vi "main.vi"() -> ()   [LabVIEW 2024]
uses:
  controls/adam-module-select-tab.ctl
  controls/digital-output-cluster.ctl
  controls/digitial-input-cluster.ctl
  controls/analog-output-cluster.ctl
  controls/analog-input-cluster.ctl
  controls/thermocouple-input-cluster.ctl
  controls/adam-5000-serial-settings.ctl
  controls/state-enum.ctl
  <vilib>/Instr/_visa.llb/VISA Configure Serial Port (Instr).vi
  <vilib>/Instr/_visa.llb/VISA Flush IO Buffer Mask.ctl
panel:
  out "response":string
  out "cmd string":string
  out "Ack":bool
  out "Sampling":bool
  in  "Module Type":T1(ring)
  out "slot: 0":T2
  in  "Digital Outputs":T3
  out "Digital Inputs":T4
  in  "Analog Outputs":T5
  out "Analog Inputs":T6
  out "Thermocouple Inputs (degC)":T7
  in  "Chassis Settings":T8={"VISA resource name"="COM10", "baud rate (19200)"=19200, "Chassis ID"=1}
  in  "Debug Mode":bool
  out "Loop Time (mS)":u32
  out "Loop Counter":i32
  out "Write Success":bool
  out "error IO":errorcluster
  out "error":errorcluster
  in  "exit":bool
  # "ADAM 5000 Controller"
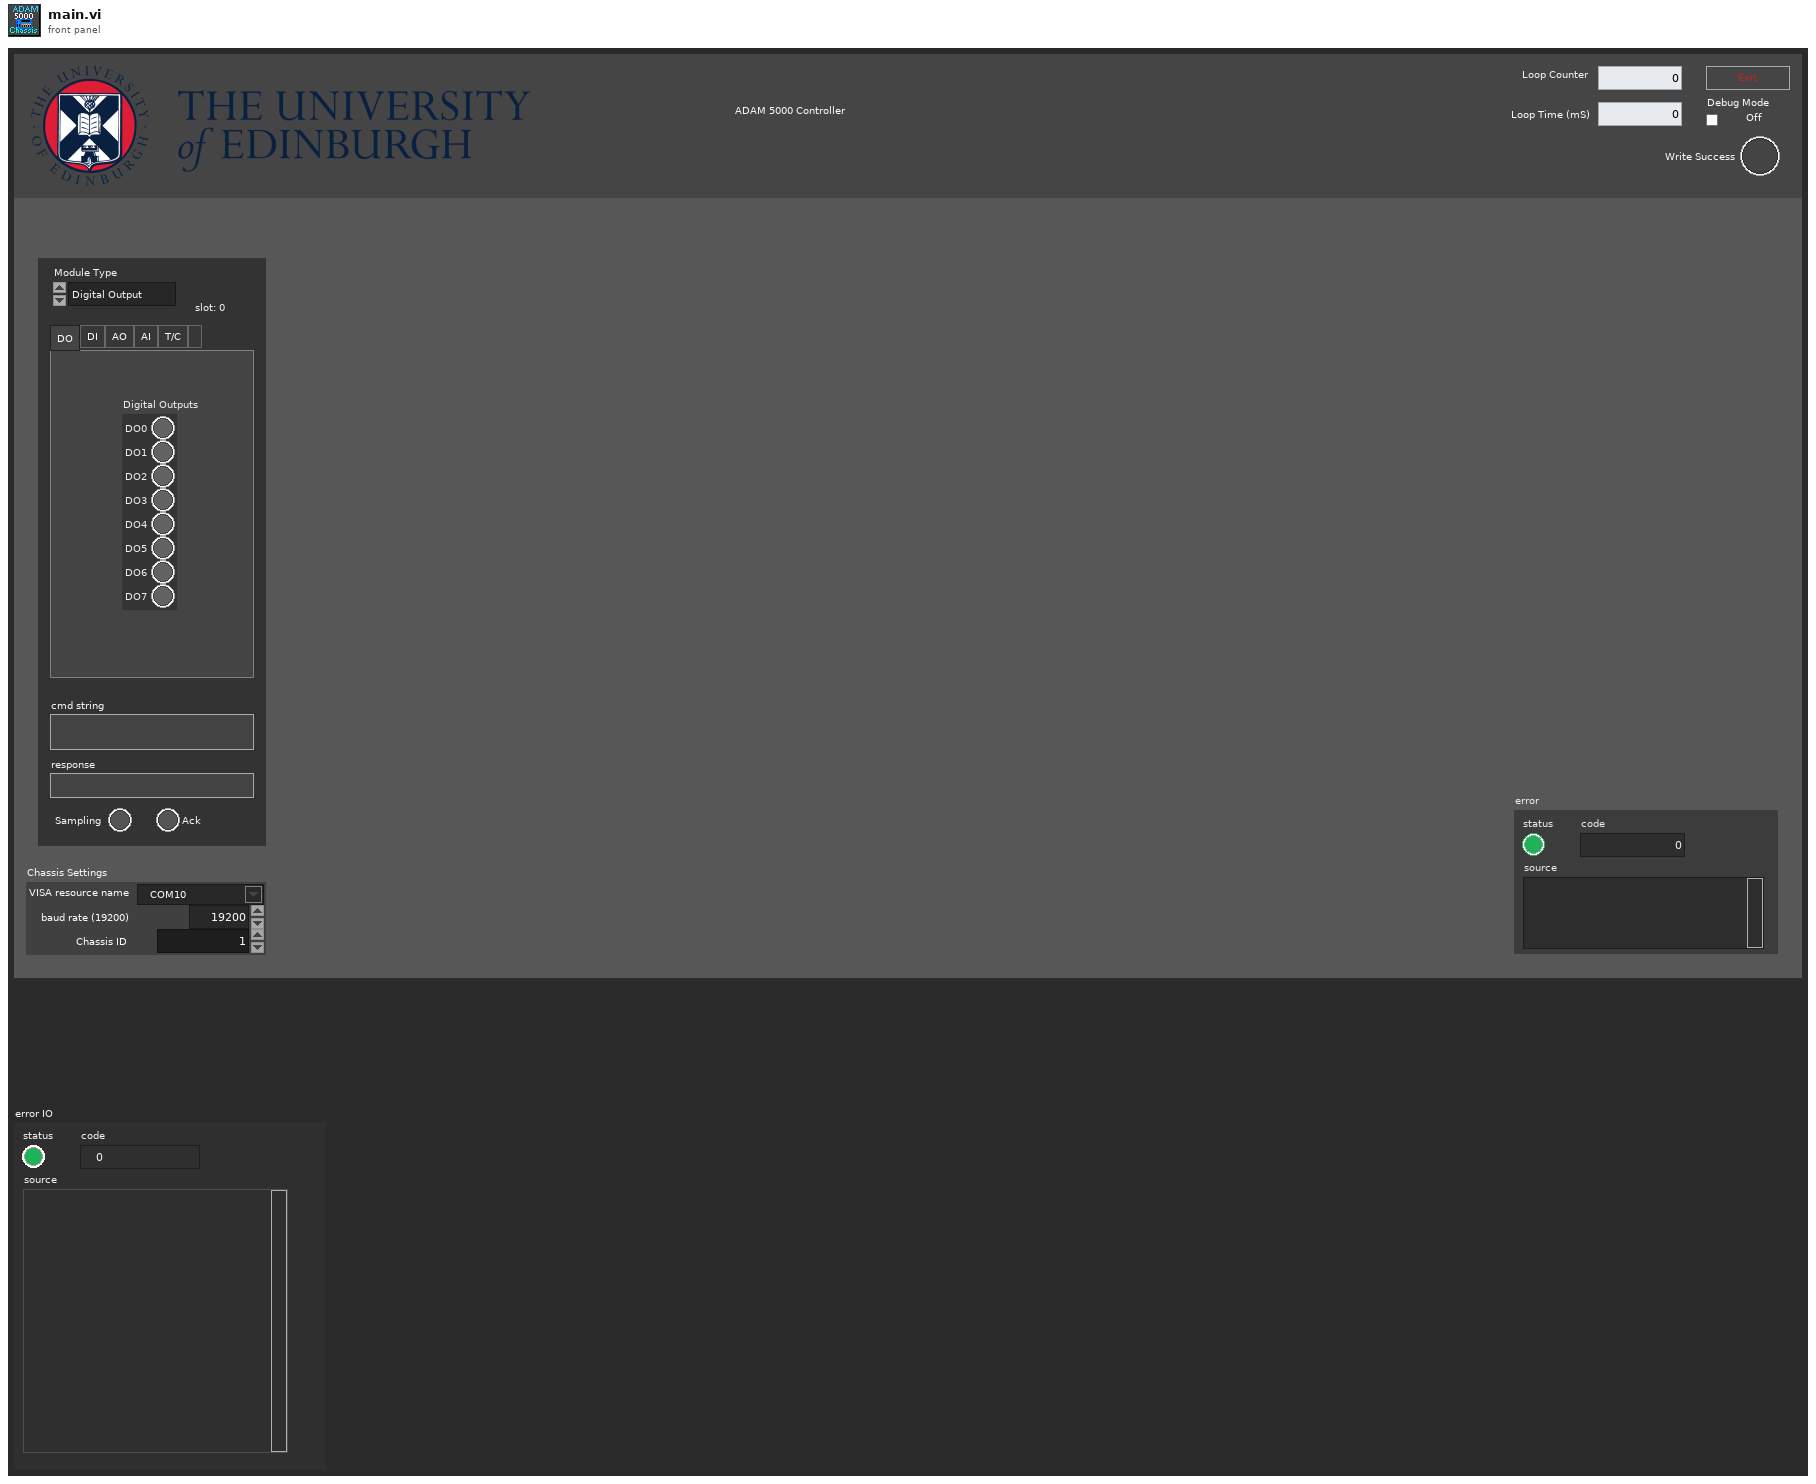
[diagram p1: front panel]
types:
  T1 = enum16{"Digital Output", "Digital Input", "Analog Output", "Analog Input", "Thermocouple", "Power Relay", "empty"}
  T2 = typedef "adam-module-select-tab.ctl" = enum32{"DO", "DI", "AO", "AI", "T/C", ""}
  T3 = typedef "digital-output-cluster.ctl" = cluster{"DO0":bool, "DO1":bool, "DO2":bool, "DO3":bool, "DO4":bool, "DO5":bool, "DO6":bool, "DO7":bool}
  T4 = typedef "digitial-input-cluster.ctl" = cluster{"DI0":bool, "DI1":bool, "DI2":bool, "DI3":bool, "DI4":bool, "DI5":bool, "DI6":bool, "DI7":bool}
  T5 = typedef "analog-output-cluster.ctl" = cluster{"AO0":dbl, "AO1":dbl, "AO2":dbl, "AO3":dbl, "AO4":dbl, "AO5":dbl, "AO6":dbl, "AO7":dbl}
  T6 = typedef "analog-input-cluster.ctl" = cluster{"AO0":dbl, "AO1":dbl, "AO2":dbl, "AO3":dbl, "AO4":dbl, "AO5":dbl, "AO6":dbl, "AO7":dbl}
  T7 = typedef "thermocouple-input-cluster.ctl" = cluster{"TC0":dbl, "TC1":dbl, "TC2":dbl, "TC3":dbl, "TC4":dbl, "TC5":dbl, "TC6":dbl}
  T8 = typedef "adam-5000-serial-settings.ctl" = cluster{"VISA resource name":refnum<visa-resource-name>, "baud rate (19200)":u32, "Chassis ID":u8}
  T9 = cluster{"Digital Outputs":T3, "Digital Inputs":T4, "Analog Outputs":T5, "Analog Inputs":T6, "Thermocouple Inputs (degC)":T7}
  T10 = typedef "state-enum.ctl" = enum16{"init", "manual", "start", "run", "hold", "stop", ""}
  T11 = typedef "VISA Flush IO Buffer Mask.ctl" = u16
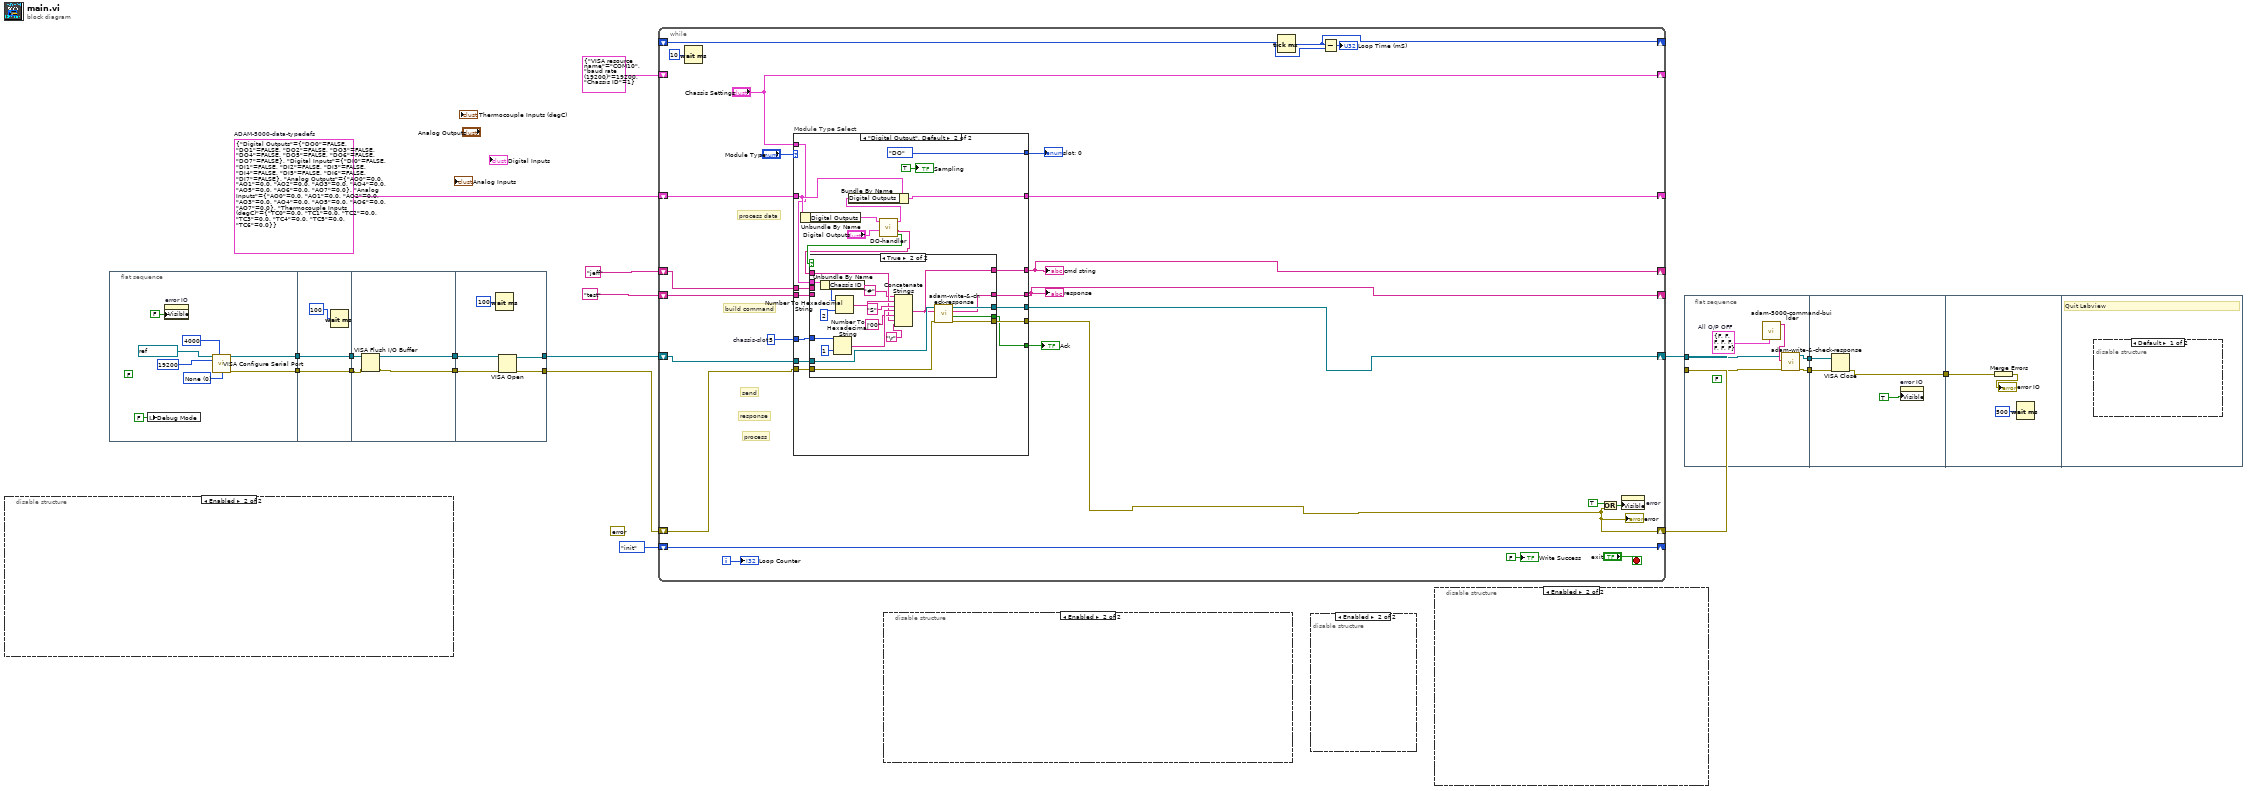
[diagram p0: block diagram]
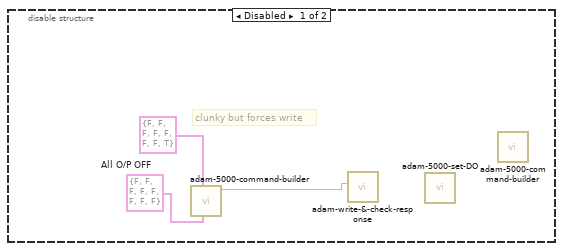
[diagram p2: hidden frame]
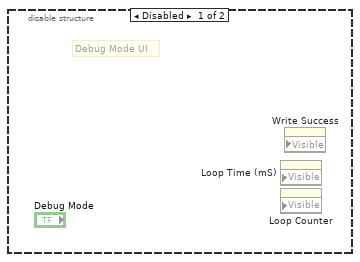
[diagram p3: hidden frame]
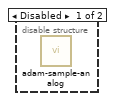
[diagram p4: hidden frame]
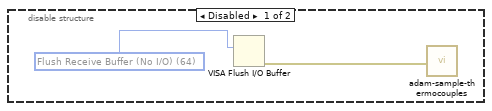
[diagram p5: hidden frame]
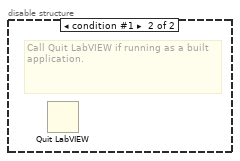
[diagram p6: hidden frame]
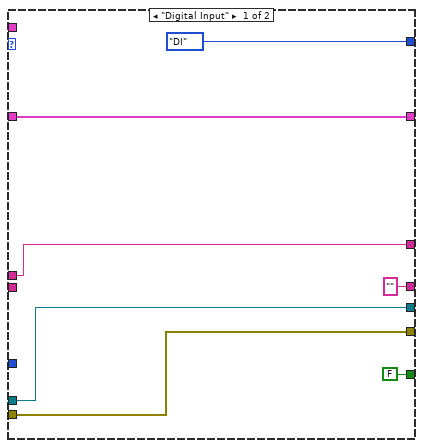
[diagram p7: hidden frame]
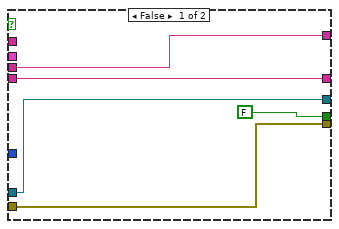
[diagram p8: hidden frame]
diagram:
  (unwired) errorcluster {"status"=FALSE, "code"=0, "source"=""} ("error")
  w13 = T9 {"Digital Outputs"={"DO0"=FALSE, "DO1"=FALSE, "DO2"=FALSE, "DO3"=FALSE, "DO4"=FALSE, "DO5"=FALSE, "DO6"=FALSE, "DO7"=FALSE}, "Digital Inputs"={"DI0"=FALSE, "DI1"=FALSE, "DI2"=FALSE, "DI3"=FALSE, "DI4"=FALSE, "DI5"=FALSE, "DI6"=FALSE, "DI7"=FALSE}, "Analog Outputs"={"AO0"=0.0, "AO1"=0.0, "AO2"=0.0, "AO3"=0.0, "AO4"=0.0, "AO5"=0.0, "AO6"=0.0, "AO7"=0.0}, "Analog Inputs"={"AO0"=0.0, "AO1"=0.0, "AO2"=0.0, "AO3"=0.0, "AO4"=0.0, "AO5"=0.0, "AO6"=0.0, "AO7"=0.0}, "Thermocouple Inputs (degC)"={"TC0"=0.0, "TC1"=0.0, "TC2"=0.0, "TC3"=0.0, "TC4"=0.0, "TC5"=0.0, "TC6"=0.0}}  # ADAM-5000-data-typedefs
  n1 = disable-structure shown="Enabled" {
    frame Disabled {
      w21 = T3 {"DO0"=FALSE, "DO1"=FALSE, "DO2"=FALSE, "DO3"=FALSE, "DO4"=FALSE, "DO5"=FALSE, "DO6"=FALSE, "DO7"=FALSE}  # All O/P OFF
      # "clunky but forces write"
      n2 = call "adam-5000-command-builder.vi"("Output Control"=w21, "Current Output State"=T3 {"DO0"=FALSE, "DO1"=FALSE, "DO2"=FALSE, "DO3"=FALSE, "DO4"=FALSE, "DO5"=FALSE, "DO6"=FALSE, "DO7"=TRUE}) -> ("Command Out"=w20:string)  [unwired: 7 in, 2 out]
      n3 = call "adam-write-&-check-response.vi"("write buffer"=w20) -> ("VISA resource name"=w19:refnum<visa-resource-name>)  [unwired: 5 in, 5 out]
      n4 = call "adam-5000-set-DO.vi"() -> ()  [unwired: 6 in, 6 out]
      n5 = call "adam-5000-command-builder.vi"() -> ()  [unwired: 9 in, 3 out]
    }
    frame Enabled {
    }
  }
  n6 = flat-sequence {
    tunnel: [w29] -> w11
    tunnel: [w28] -> w10
    tunnel: w11 -> [w33]
    tunnel: [w33] -> w9
    tunnel: w10 -> [w32]
    tunnel: [w32] -> w8
    tunnel: w9 -> [w37]
    tunnel: [w35] -> w7
    tunnel: w8 -> [w36]
    tunnel: [w34] -> w6
    tunnel: w7 -> [w41]
    tunnel: w6 -> [w40]
    tunnel: [w39] -> w5
    tunnel: [w38] -> w4
    frame #0 {
      w26 = u16 0 items=["None", "XON/XOFF", "RTS/CTS", "XON/XOFF & RTS/CTS", "DTR/DSR", "XON/XOFF & DTR/DSR"] ("flow control (0:none)")
      (unwired) FALSE ("V1")
      n7 = local write "Debug Mode"(FALSE ("Debug Mode")) -> ()
      n8 = property on="error IO" class="Clust (strict)"("Visible"=FALSE) -> ()  [unwired: 2 in, 2 out]
      n9 = call-poly "VISA Configure Serial Port"("VISA resource name"=refnum<visa-resource-name> "COM10", "timeout (10sec)"=u32 4000, "baud rate (9600)"=u32 19200, "flow control (0:none)"=w26) -> ("VISA resource name out"=w29:refnum<visa-resource-name>, "error out"=w28:errorcluster)  [unwired: 10 in]
    }
    frame #1 {
      n10 = Wait (ms)(milliseconds to wait=u32 100) -> ()  [unwired: 1 out]
    }
    frame #2 {
      n11 = VISA Flush I/O Buffer(VISA resource name=w37, error in (no error)=w36) -> (VISA resource name out=w35:refnum<visa-resource-name>, error out=w34:errorcluster)  [unwired: 1 in]
    }
    frame #3 {
      n12 = Wait (ms)(milliseconds to wait=u32 100) -> ()  [unwired: 1 out]
      n13 = VISA Open(error in (no error)=w40, VISA resource name=w41) -> (VISA resource name=w39:refnum<visa-resource-name>, error out=w38:errorcluster)  [unwired: 3 in]
    }
  }
  n14 = while {
    shift-right: [w59] -> _
    shift-left: state-enum."init" ("state-enum") -> [w59]
    shift-right: [w50] -> w17
    shift-left: w4 -> [w51]
    shift-right: [w62] -> _
    shift-left: _ -> [w64]
    shift-right: [w54] -> _
    shift-left: w13 -> [w57]
    shift-right: ["Chassis Settings"] -> _
    shift-left: T8 {"VISA resource name"="COM10", "baud rate (19200)"=19200, "Chassis ID"=1} ("Chassis Settings") -> [_]
    shift-right: [w49] -> w3
    shift-left: w5 -> [w52]
    shift-right: [w48] -> _
    shift-left: "test" ("acknowledge char") -> [w47]
    shift-right: [w45] -> _
    shift-left: "jeff" -> [w44]
    i -> [w65]
    stop <- "exit" stop-if-true
    w53 = 5  # chassis-slot
    # "process"
    # "response"
    # "send"
    # "build command"
    # "process data"
    n15 = Wait (ms)(milliseconds to wait=u32 10) -> ()  [unwired: 1 out]
    n16 = case "Module Type Select" shown="\"Digital Output\", Default" "Module Type" {
      tunnel: w57 -> [w73 w90]
      tunnel: [adam-module-select-tab."DI" ("slot: 0") adam-module-select-tab."DO" ("slot: 0")] -> w55
      tunnel: [w73 w91] -> w54
      tunnel: "Chassis Settings" -> [_ w86]
      tunnel: w53 -> [_ w85]
      tunnel: w52 -> [w72 w84]
      tunnel: w51 -> [w71 w83]
      tunnel: [w71 w82] -> w50
      tunnel: [w72 w81] -> w49
      tunnel: ["" ("acknowledge char") w79] -> w48
      tunnel: w47 -> [_ w78]
      tunnel: [FALSE ("cmd aknowledged") w77] -> w46
      tunnel: [w68 w76] -> w45
      tunnel: w44 -> [w68 w75]
      frame "Digital Input" {
      }
      frame "Digital Output", Default {
        n17 = Unbundle By Name(w90) -> ("Digital Outputs"=w93:T3)
        n18 = call "DO-handler.vi"("Output Control"="Digital Outputs", "Current Output State"=w93) -> ("output state changed"=w88:bool, "hex integer string"=w87:string, "DO Output"=w89:T3)  [unwired: 5 in, 2 out]
        n19 = case shown="True" w88 {
          tunnel: w87 -> [_ w109]
          tunnel: w86 -> [_ w118]
          tunnel: w85 -> [_ w113]
          tunnel: w84 -> [w99 w107]
          tunnel: w83 -> [w97 w106]
          tunnel: [w97 w105] -> w82
          tunnel: [w99 w104] -> w81
          tunnel: [FALSE ("cmd aknowledged") w103] -> w77
          tunnel: [w96 w102] -> w79
          tunnel: w78 -> [w96 _]
          tunnel: [w95 w101] -> w76
          tunnel: w75 -> [w95 _]
          frame False {
          }
          frame True {
            n20 = Unbundle By Name(w118) -> ("Chassis ID"=w117:u8)
            n21 = Number To Hexadecimal String(1:i16 1 ("width (-)"), 2:w113) -> (0:w111:string)
            n22 = Number To Hexadecimal String(1:i16 2 ("width (-)"), 2:w117) -> (0:w115:string)
            n23 = Concatenate Strings("#" ("string"), w115, "S" ("string"), w111, "00" ("string"), w109, "\r") -> (w101:string)
            n24 = call "adam-write-&-check-response.vi"("error in (no error)"=w106, "write buffer"=w101, "VISA resource name"=w107) -> ("error out"=w105:errorcluster, "cmd aknowledged"=w103:bool, "acknowledge char"=w102:string, "VISA resource name out"=w104:refnum<visa-resource-name>)  [unwired: 4 in, 1 out]
          }
        }
        n25 = Bundle By Name(cluster=w90, "Digital Outputs"=w89) -> (w91:T9)
        "Sampling" <- TRUE ("Sampling")
      }
    }
    "error" <- w50
    "slot: 0" <- w55
    "response" <- w48
    "Ack" <- w46
    "cmd string" <- w45
    n26 = Tick Count (ms)() -> (millisecond timer value=w62:u32)
    n27 = Subtract(x=w62, y=w64) -> (x-y=→"Loop Time (mS)":u32)
    n28 = Or(x=TRUE ("Debug Mode"), y=w50) -> (x .or. y?=w61:bool)
    n29 = property on="error" class="Clust (strict)"("Visible"=w61) -> ()  [unwired: 2 in, 2 out]
    "Write Success" <- FALSE ("Write Success")
    "Loop Counter" <- w65
  }
  n30 = disable-structure shown="Enabled" {
    frame Disabled {
      w123 = T11 64 items=["Flush Receive Buffer"=16, "Write Transmit Buffer to Device"=32, "Flush Receive Buffer (No I/O)"=64, "Flush Transmit Buffer"=128] ("Mask")
      n31 = VISA Flush I/O Buffer(mask (16)=w123) -> (error out=w122:errorcluster)  [unwired: 2 in, 1 out]
      n32 = call "adam-sample-thermocouples.vi"("error in (no error)"=w122) -> ("status"=w120:string, "read buffer"=w119:string, "acknowledge char"=w121:string)  [unwired: 5 in, 3 out]
    }
    frame Enabled {
    }
  }
  n33 = disable-structure shown="Enabled" {
    frame Disabled {
      n34 = call "adam-sample-analog.vi"() -> ()  [unwired: 6 in, 6 out]
    }
    frame Enabled {
    }
  }
  n35 = disable-structure shown="Enabled" {
    frame Disabled {
      # "Debug Mode UI"
      n36 = property on="Loop Time (mS)" class="DigNum (strict)" props=["Visible"]() -> ()  [unwired: 3 in, 2 out]
      n37 = property on="Loop Counter" class="DigNum (strict)" props=["Visible"]() -> ()  [unwired: 3 in, 2 out]
      n38 = property on="Write Success" class="Bool (strict)" props=["Visible"]() -> ()  [unwired: 3 in, 2 out]
    }
    frame Enabled {
    }
  }
  n39 = flat-sequence {
    tunnel: w17 -> [w129]
    tunnel: [w128] -> w15
    tunnel: [w127] -> w14
    tunnel: w3 -> [w125]
    tunnel: [w131] -> w16
    tunnel: w15 -> [w132]
    tunnel: w14 -> [w133]
    tunnel: w16 -> [w135]
    frame #0 {
      (unwired) FALSE ("V1")
      w126 = T3 {"DO0"=FALSE, "DO1"=FALSE, "DO2"=FALSE, "DO3"=FALSE, "DO4"=FALSE, "DO5"=FALSE, "DO6"=FALSE, "DO7"=FALSE}  # All O/P OFF
      n40 = call "adam-5000-command-builder.vi"("Output Control"=w126) -> ("Command Out"=w130:string)  [unwired: 8 in, 2 out]
      n41 = call "adam-write-&-check-response.vi"("error in (no error)"=w129, "write buffer"=w130, "VISA resource name"=w125) -> ("error out"=w127:errorcluster, "VISA resource name out"=w128:refnum<visa-resource-name>)  [unwired: 4 in, 3 out]
    }
    frame #1 {
      n42 = VISA Close(VISA resource name=w132, error in (no error)=w133) -> (error out=w131:errorcluster)
      n43 = property on="error IO" class="Clust (strict)"("Visible"=TRUE) -> ()  [unwired: 2 in, 2 out]
    }
    frame #2 {
      n44 = Merge Errors(w135) -> (→"error IO":errorcluster)
      n45 = Wait (ms)(milliseconds to wait=u32 500) -> ()  [unwired: 1 out]
    }
    frame #3 {
      # "Quit Labview"
      n46 = disable-structure "Conditional Disable Structure" shown="Default" {
        frame condition #0 (active) {
        }
        frame condition #1 {
          # "Call Quit LabVIEW if running as a built application."
          n47 = Quit LabVIEW() -> ()  [unwired: 1 in]
        }
      }
    }
  }
